vi "Modbus Master2.vi"() -> ()   [LabVIEW 2015]
uses:
  <vilib>/Modbus/master/Create Master Instance (Serial).vi
  <vilib>/Modbus/master/Modbus Master.lvclass
panel:
  in  "SV":u16
  out "SV":dbl
  out "PV":dbl
  out "register values":u16[](array[numeric])
  in  "stop":bool
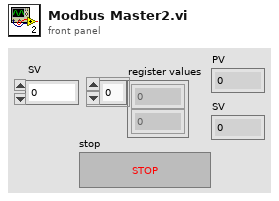
[diagram p1: front panel]
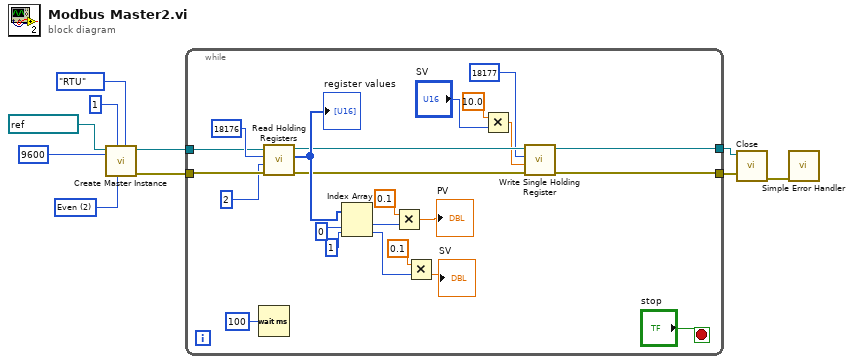
[diagram p0: block diagram]
diagram:
  w7 = u16 2 items=["None", "Odd", "Even"] ("parity (Even)")
  n1 = call-poly <vilib>:"Create Master Instance.vi"("serial type"=enum16{"RTU", "ASCII"}."RTU", "parity (Even)"=w7, "unit ID"=u8 1, "baud rate (9600)"=u32 9600, "VISA resource name"=refnum<visa-resource-name> "COM5") -> ("error out"=w4:errorcluster, "serial master instance"=w2:refnum<class "Modbus Master.lvclass">)  [unwired: 5 in]
  n2 = while {
    tunnel: w4 -> [w32]
    tunnel: [w23] -> w3
    tunnel: w2 -> [w28]
    tunnel: [w21] -> w1
    stop <- "stop" stop-if-true
    n3 = Wait (ms)(milliseconds to wait=u32 100) -> ()  [unwired: 1 out]
    n4 = call-dynamic "Read Holding Registers.vi"("error in (no error)"=w32, "number of holding registers"=u16 2, "starting address"=u16 18176, "Modbus master in"=w28) -> ("error out"=w24:errorcluster, "register values"=w27:u16[], "Modbus master out"=w22:refnum<class "Modbus Master.lvclass">)  [unwired: 5 in]
    "register values" <- w27
    n5 = Index Array(array=w27, index #1=0 ("index"), index #2=1 ("index")) -> (element #1=w19:u16, element #2=w16:u16)
    n6 = Multiply(x=0.1, y=w19) -> (x*y=→"PV":dbl)
    n7 = Multiply(x=0.1, y=w16) -> (x*y=→"SV":dbl)
    n8 = Multiply(x=10.0, y="SV") -> (x*y=w12:dbl)
    n9 = call-dynamic "Write Single Holding Register.vi"("error in (no error)"=w24, "holding register value"=w12, "address"=u16 18177 ("starting address"), "Modbus master in"=w22) -> ("error out"=w23:errorcluster, "Modbus master out"=w21:refnum<class "Modbus Master.lvclass">)  [unwired: 6 in]
  }
  n10 = call-dynamic "Close.vi"("error in (no error)"=w3, "Modbus master in"=w1) -> ("error out"=w5:errorcluster)  [unwired: 9 in]
  n11 = call <vilib>:"Simple Error Handler.vi"("error in (no error)"=w5) -> ()  [unwired: 4 in, 5 out]
